vi "WS1050 Stress RB REG.vi"(8 "error in (no error)":errorcluster, 11 "Set RB REG":string[](array[string])) -> (0 "error out":errorcluster, 3 "Data out":string[](array[string]))   [LabVIEW 2012]
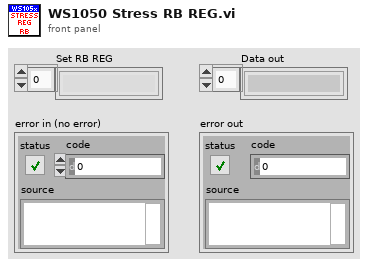
[diagram p1: front panel]
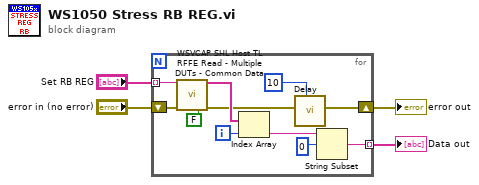
[diagram p0: block diagram]
diagram:
  n1 = for {
    tunnel: "Set RB REG" -> [w15] mode=indexing
    tunnel: [w11] -> w4 mode=indexing
    shift-right: [w8] -> w1
    shift-left: "error in (no error)" -> [w14]
    i -> [w13]
    n2 = call "WSVCAP SHL Host TL RFFE Read - Multiple DUTs - Common Data.vi"("Data Out"=w15, "error in"=w14, "Log (T)"=FALSE) -> ("RFFE Data In"=w10:string[], "error out"=w7:errorcluster)  [unwired: 11 in]
    n3 = Index Array(array=w10, index=w13) -> (element=w9:string)
    n4 = call "Delay.vi"("milliseconds to wait"=u32 10, "error in (no error)"=w7) -> ("error out"=w8:errorcluster)  [unwired: 9 in]
    n5 = String Subset(string=w9, offset (0)=0) -> (substring=w11:string)  [unwired: 1 in]
  }
  "Data out" <- w4
  "error out" <- w1
